vi "ErrorCtrlFormater.vi"(8 "error in (no error)":errorcluster, 11 "Control in":refnum<vi>) -> (0 "error out":errorcluster, 3 "Changed":bool)   [LabVIEW 2017]
uses:
  <vilib>/Utility/miscctls.llb/LVBoundsTypeDef.ctl
  <vilib>/Utility/miscctls.llb/LVPositionTypeDef.ctl
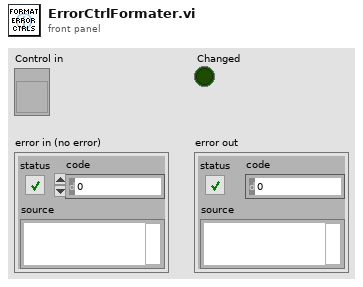
[diagram p1: front panel]
types:
  T1 = typedef "LVPositionTypeDef.ctl" = cluster{"Left":i32, "Top":i32}
  T2 = typedef "LVBoundsTypeDef.ctl" = cluster{"Width":u32, "Height":u32}
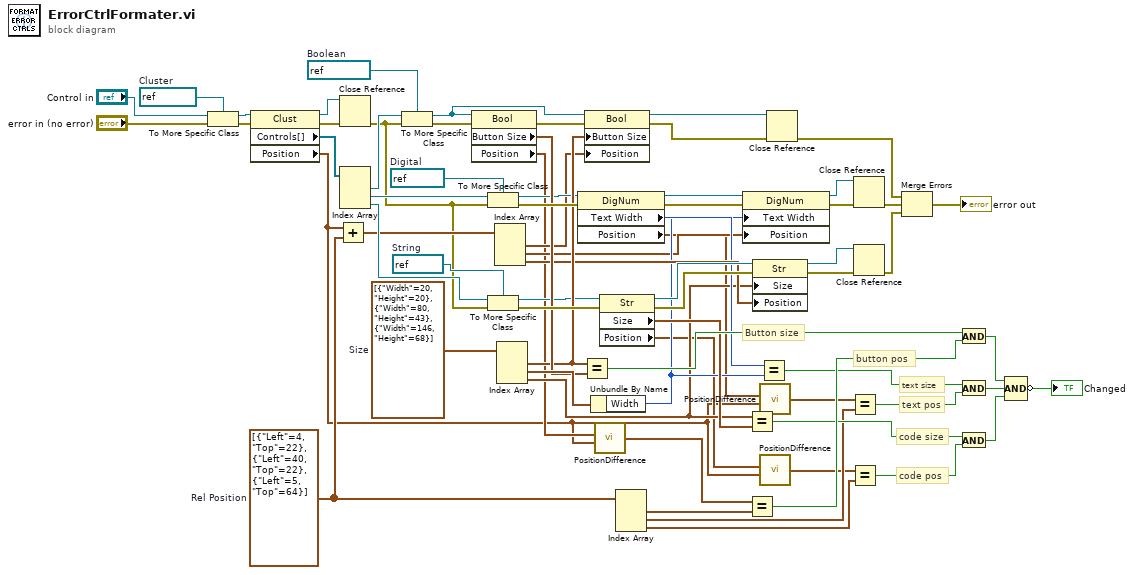
[diagram p0: block diagram]
diagram:
  w8 = T1[] [{"Left"=4, "Top"=22}, {"Left"=40, "Top"=22}, {"Left"=5, "Top"=64}]  # Rel Position
  w54 = T2[] [{"Width"=20, "Height"=20}, {"Width"=80, "Height"=43}, {"Width"=146, "Height"=68}]  # Size
  w62 = refnum<vi> refnum  # String
  w63 = refnum<vi> refnum  # Boolean
  w64 = refnum<vi> refnum  # Digital
  w68 = refnum<vi> refnum  # Cluster
  # "button pos"
  # "text pos"
  # "code size"
  # "code pos"
  # "text size"
  # "Button size"
  n1 = To More Specific Class(target class=w68, reference="Control in", error in="error in (no error)") -> (specific class reference=w66:refnum<vi>, error out=w65:errorcluster)
  n2 = property class="Clust"(reference=w66, error in=w65) -> (reference out=w43:refnum<vi>, error out=w42:errorcluster, "Controls[]"=w61:refnum<vi>[], "Position"=w2:T1)
  n3 = Add(x=w2, y=w8) -> (x+y=w53:T1[])
  n4 = Close Reference(reference=w43, error in (no error)=w42) -> (error out=w41:errorcluster)
  n5 = Index Array(array=w61) -> (element #1=w60:refnum<vi>, element #2=w59:refnum<vi>, element #3=w58:refnum<vi>)  [unwired: 3 in]
  n6 = To More Specific Class(target class=w63, reference=w60, error in=w41) -> (specific class reference=w39:refnum<vi>, error out=w38:errorcluster)
  n7 = property class="Bool"(reference=w39, error in=w38) -> (error out=w37:errorcluster, "Button Size"=w36:T2, "Position"=w4:T1)  [unwired: 1 out]
  n8 = To More Specific Class(target class=w64, reference=w59, error in=w41) -> (specific class reference=w24:refnum<vi>, error out=w56:errorcluster)
  n9 = To More Specific Class(target class=w62, reference=w58, error in=w41) -> (specific class reference=w31:refnum<vi>, error out=w55:errorcluster)
  n10 = Index Array(array=w53) -> (element #1=w9:T1, element #2=w20:T1, element #3=w28:T1)  [unwired: 3 in]
  n11 = Index Array(array=w54) -> (element #1=w35:T2, element #2=w40:T2, element #3=w11:T2)  [unwired: 3 in]
  n12 = property class="DigNum"(reference=w24, error in=w56) -> (reference out=w23:refnum<vi>, error out=w25:errorcluster, "Text Width"=w22:u32, "Position"=w1:T1)
  n13 = Equal?(x=w35, y=w36) -> (x = y?=w33:bool)
  n14 = property class="Bool"(reference=w39, error in=w37, "Button Size"=w35, "Position"=w9) -> (reference out=w51:refnum<vi>, error out=w52:errorcluster)
  n15 = Unbundle By Name(w40) -> ("Width"=w21:u32)
  n16 = call "PositionDifference.vi"("(x,y)"=w4, "(x1,y1)"=w2) -> ("(x-x1,y-y1)"=w5:T1)  [unwired: 3 in]
  n17 = property class="Str"(reference=w31, error in=w55) -> (reference out=w30:refnum<vi>, error out=w32:errorcluster, "Size"=w29:T2, "Position"=w7:T1)
  n18 = Index Array(array=w8) -> (element #1=w12:T1, element #2=w13:T1, element #3=w10:T1)  [unwired: 3 in]
  n19 = property class="DigNum"(reference=w23, error in=w25, "Text Width"=w21, "Position"=w20) -> (reference out=w48:refnum<vi>, error out=w49:errorcluster)
  n20 = Equal?(x=w11, y=w29) -> (x = y?=w27:bool)
  n21 = Equal?(x=w5, y=w12) -> (x = y?=w34:bool)
  n22 = property class="Str"(reference=w30, error in=w32, "Size"=w11, "Position"=w28) -> (reference out=w45:refnum<vi>, error out=w46:errorcluster)
  n23 = Equal?(x=w22, y=w21) -> (x = y?=w19:bool)
  n24 = call "PositionDifference.vi"("(x,y)"=w1, "(x1,y1)"=w2) -> ("(x-x1,y-y1)"=w3:T1)  [unwired: 3 in]
  n25 = call "PositionDifference.vi"("(x,y)"=w7, "(x1,y1)"=w2) -> ("(x-x1,y-y1)"=w6:T1)  [unwired: 3 in]
  n26 = Close Reference(reference=w51, error in (no error)=w52) -> (error out=w50:errorcluster)
  n27 = Equal?(x=w3, y=w13) -> (x = y?=w18:bool)
  n28 = Equal?(x=w6, y=w10) -> (x = y?=w26:bool)
  n29 = Close Reference(reference=w48, error in (no error)=w49) -> (error out=w47:errorcluster)
  n30 = Close Reference(reference=w45, error in (no error)=w46) -> (error out=w44:errorcluster)
  n31 = Merge Errors(w50, w47, w44) -> (→"error out":errorcluster)
  n32 = And(x=w33, y=w34) -> (x .and. y?=w17:bool)
  n33 = And(x=w19, y=w18) -> (x .and. y?=w16:bool)
  n34 = And(x=w27, y=w26) -> (x .and. y?=w15:bool)
  n35 = Compound Arithmetic op=AND(w17, w16, w15) -> (invert →"Changed":bool)
